vi "CHD_DRIVE_EXECUTE.vi"(6 "Pass_Through_Time":dbl=-1.0 format="%33.4f", 8 "error in (no error)":errorcluster) -> (0 "error out":errorcluster)   [LabVIEW 2019]
uses:
  <vilib>/Rock Robotics/WPI/ThirdParty/JAS_Junk/TrajLib/VI/BoolCmd_Recv_Internal.vi
  <vilib>/Rock Robotics/WPI/ThirdParty/JAS_Junk/TrajLib/VI/numCmd_Recv_Generic.vi
  <vilib>/Rock Robotics/WPI/ThirdParty/JAS_Junk/TrajLib/VI/Util_GetTime_U32.vi
  <vilib>/Rock Robotics/WPI/ThirdParty/JAS_Junk/TrajLib/MathUtil_InputModulus.vi
  <vilib>/Rock Robotics/WPI/ThirdParty/JAS_Junk/TrajLib/VI/BoolCmd_ObtainQueue.vi
  <vilib>/Rock Robotics/WPI/ThirdParty/JAS_Junk/TrajLib/VI/numCmd_ObtainQueue_Generic.vi
  CHD_DRIVE_GLOBALS.vi
  <vilib>/Rock Robotics/SystemInterfaces/Utilities/FPGA_UtilitiesRead LocalTime.vi
  <vilib>/Rock Robotics/WPI/ThirdParty/JAS_Junk/TrajLib/VI/Util_GetTime_U64.vi
  <vilib>/Rock Robotics/WPI/ThirdParty/JAS_Junk/TrajLib/Trajectory_Library.lvlib
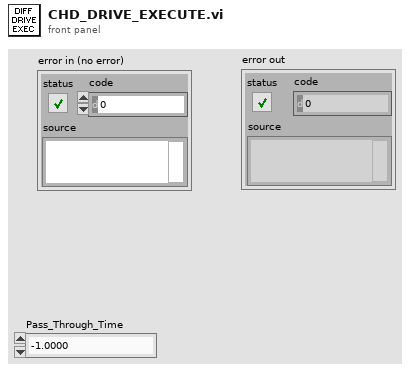
[diagram p1: front panel]
types:
  T1 = typedef "WPI_GyroDevRef.ctl" = cluster{"DevStatus":errorcluster, "Analog Channel":T2, "Gain (VoltsPerDegree/Second)":dbl, "Gyro Type":enum16{"Analog", "XRS450"}, "Handle":i32, "SPI Bus":T3, "Device Found":bool, "Sample Rate":dbl, "Calibrate On Open":bool, "Offset":dbl}
  T2 = typedef "FPGA_AIChannel.ctl" = enum8{"AI 0", "AI 1", "AI 2", "AI 3", "AI MXP 0", "AI MXP 1", "AI MXP 2", "AI MXP 3", "Invalid"}
  T3 = typedef "spi_bus.ctl" = enum16{"SPI On-Board, CS0", "SPI On-Board, CS1", "SPI On-Board, CS2", "SPI On-Board, CS3", "SPI MXP", "Invalid"}
  T4 = typedef "CHD_DRIVE_MODULE_TYPDEF.ctl" = cluster{"DiffDriveMotor":T5, "DiffDriveEnc":T10}
  T5 = typedef "WPI_MotorControlDeviceRef.ctl" = cluster{"DeviceStatus":errorcluster, "Type":T6, "PWM":cluster{"PWM Channel":T7, "DeadBand":T8}, "CAN":cluster{"Device Number":u8, "SetOutput VI Ref":variant, "GetOutput VI Ref":variant, "Enable VI Ref":variant, "Disable VI Ref":variant, "Data":variant}, "Invert":bool, "DIO PWM":cluster{"PWM \"Enable\" Channel":T7, "DIOChannel":T9, "PWM Rate":dbl}}
  T6 = typedef "WPI_MotorControlType.ctl" = enum16{"PWM", "CAN", "DIO PWM"}
  T7 = typedef "FPGA_DIOPWMChannel.ctl" = enum8{"PWM 0", "PWM 1", "PWM 2", "PWM 3", "PWM 4", "PWM 5", "PWM 6", "PWM 7", "PWM 8", "PWM 9", "PWM MXP 0", "PWM MXP 1", "PWM MXP 2", "PWM MXP 3", "PWM MXP 4", "PWM MXP 5", "PWM MXP 6", "PWM MXP 7", "PWM MXP 8", "PWM MXP 9", "Invalid"}
  T8 = typedef "WPI_PWMDeadband.ctl" = cluster{"Name":string, "maxPositivePwm":i32, "minPositivePwm":i32, "centerPwm":i32, "maxNegativePwm":i32, "minNegativePwm":i32, "angularRange":u16}
  T9 = typedef "FPGA_DIOChannel.ctl" = enum8{"DIO 0", "DIO 1", "DIO 2", "DIO 3", "DIO 4", "DIO 5", "DIO 6", "DIO 7", "DIO 8", "DIO 9", "DIO MXP 0", "DIO MXP 1", "DIO MXP 2", "DIO MXP 3", "DIO MXP 4", "DIO MXP 5", "DIO MXP 6", "DIO MXP 7", "DIO MXP 8", "DIO MXP 9", "DIO MXP 10", "DIO MXP 11", "DIO MXP 12", "DIO MXP 13", "DIO MXP 14", "DIO MXP 15", "SPI Port CS1", "SPI Port CS2", "SPI Port CS3", "SPI Port MISO", "SPI Port MOSI", "Invalid"}
  T10 = typedef "WPI_EncoderDevRef.ctl" = cluster{"DevStatus":errorcluster, "EncoderIndex":T11, "CounterIndex":T12, "DistancePerCount":dbl, "Decoding Type":T13}
  T11 = typedef "FPGA_EncoderIdx.ctl" = enum8{"Enc 0", "Enc 1", "Enc 2", "Enc 3", "Enc 4", "Enc 5", "Enc 6", "Enc 7", "Invalid"}
  T12 = typedef "FPGA_CounterCtrSystemIndex.ctl" = enum8{"Ctr 0", "Ctr 1", "Ctr 2", "Ctr 3", "Ctr 4", "Ctr 5", "Ctr 6", "Ctr 7", "Invalid"}
  T13 = typedef "WPI_EncoderType.ctl" = enum16{"1x", "2x", "4x"}
  T14 = typedef "Trajectory_Library.lvlib/DIFF_DRIVE_KINEMATICS.ctl" = cluster{"TrackWidth_Meters":dbl}
  T15 = typedef "Trajectory_Library.lvlib/CHASSIS_SPEEDS.ctl" = cluster{"vX":dbl, "vY":dbl, "vOmega":dbl}
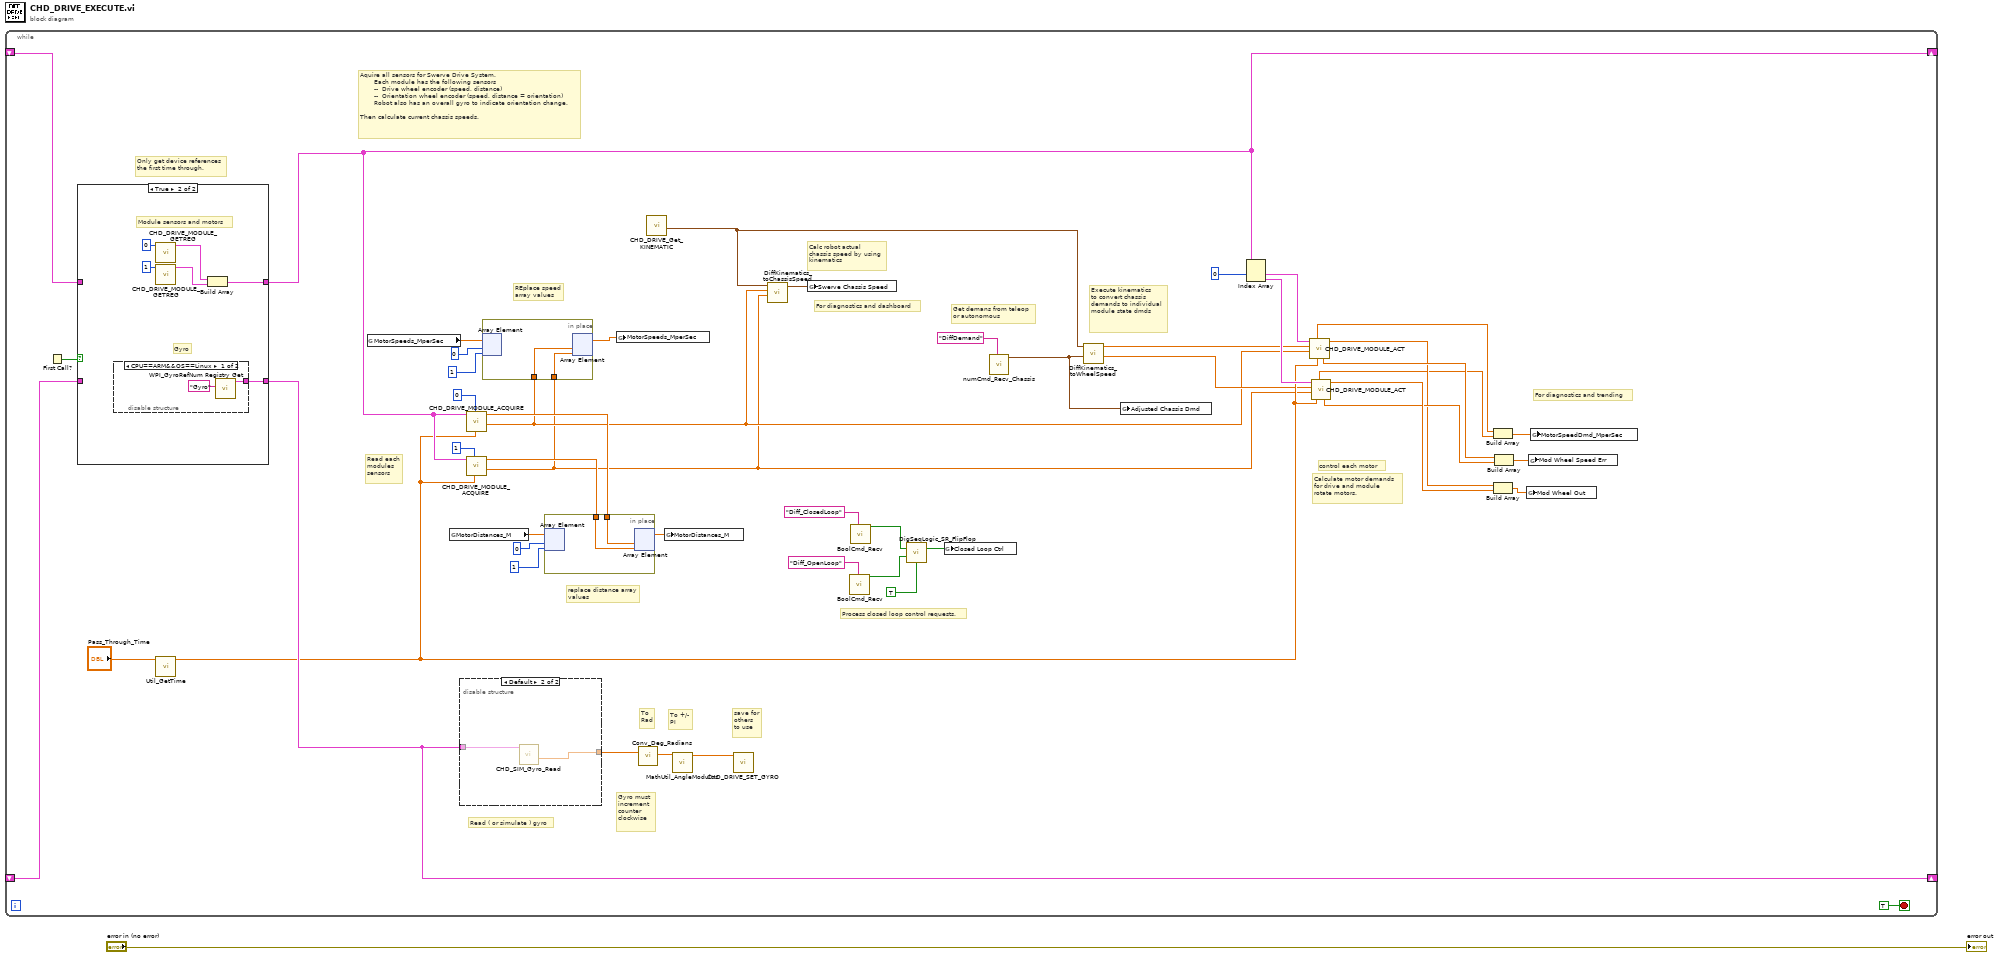
[diagram p0: block diagram]
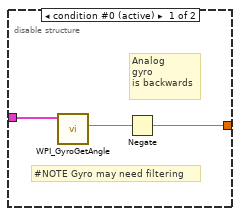
[diagram p4: hidden frame]
diagram:
  n1 = while {
    shift-right: [w29] -> _
    shift-left: _ -> [w30]
    shift-right: [w28] -> _
    shift-left: _ -> [w27]
    stop <- TRUE stop-if-true
    # "replace distance array\nvalues"
    # "REplace speed\narray values"
    # "Process closed loop control requests."
    # "Only get device references\nthe first time through."
    # "save for\nothers\nto use"
    # "For diagnostics and trending"
    # "For diagnostics and dashboard"
    # "Read each\nmodules\nsensors"
    # "Gyro must\nincrement \ncounter\nclockwise"
    # "To +/-\nPI"
    # "To\nRad"
    # "Read ( or simulate ) gyro"
    # "Aquire all sensors for Swerve Drive System.\n       Each module has the following sensors\n       --  Drive wheel encoder (speed, distance)\n       --  Orientation wheel encoder (speed, distance = orientation)\n       Robot also has an overall gyro to indicate orientation change.\n\nThen calculate current chassis speeds."
    # "Calc robot actual\nchassis speed by using\nkinematics"
    # "Calculate motor demands\nfor drive and module \nrotate motors."
    # "Execute kinematics\nto convert chassis \ndemands to individual\nmodule state dmds"
    # "Get demans from teleop\nor autonomous"
    # "control each motor"
    n2 = First Call?() -> (First Call?: T/F=w31:bool)
    n3 = case shown="True" w31 {
      tunnel: [w56 w60] -> w29
      tunnel: [w55 w59] -> w28
      tunnel: w30 -> [w56 _]
      tunnel: w27 -> [w55 _]
      frame False {
      }
      frame True {
        # "Module sensors and motors"
        # "Gyro"
        n4 = disable-structure shown="CPU==ARM&&OS==Linux" {
          disable-tunnel: [w63 _] -> w59
          frame condition #0 (active) {
            n5 = call <vilib>:"WPI_GyroRefNum Registry Get.vi"("refnum name"="Gyro") -> ("GyroDevRef"=w63:T1)  [unwired: 9 in, 1 out]
          }
          frame condition #1 {
          }
        }
        n6 = call "CHD_DRIVE_MODULE_GETREG.vi"("Suffix"=0) -> ("Diff Module TypDef"=w61:T4)  [unwired: 10 in]
        n7 = call "CHD_DRIVE_MODULE_GETREG.vi"("Suffix"=1) -> ("Diff Module TypDef"=w62:T4)  [unwired: 10 in]
        n8 = Build Array(w61, w62) -> (w60:T4[])
      }
    }
    n9 = call <vilib>:"Util_GetTime.vi"("Pass_Through_Time"="Pass_Through_Time") -> ("FPGA_Time_Seconds"=w17:dbl)  [unwired: 8 in, 2 out]
    n10 = global read "CHD_DRIVE_GLOBALS.vi" "MotorSpeeds_MperSec"() -> (w9:dbl[])
    n11 = global read "CHD_DRIVE_GLOBALS.vi" "MotorDistances_M"() -> (w6:dbl[])
    n12 = disable-structure shown="Default" {
      disable-tunnel: w28 -> [w67 w69]
      disable-tunnel: [w65 w68] -> w35
      frame condition #0 (active) {
        # "Analog\ngyro\nis backwards"
        # "#NOTE Gyro may need filtering"
        n13 = call <vilib>:"WPI_GyroGetAngle.vi"("GyroDevRef"=w67) -> ("Angle"=w66:dbl)  [unwired: 6 in, 4 out]
        n14 = Negate(x=w66) -> (-x=w65:dbl)
      }
      frame condition #1 {
        n15 = call "CHD_SIM_Gyro_Read.vi"("GyroDevRef"=w69) -> ("Gyro_Cont_Deg"=w68:dbl)  [unwired: 10 in]
      }
    }
    n16 = call "CHD_DRIVE_MODULE_ACQUIRE.vi"("Pass_Through_Time"=w17, "Swerve Module Inx"=1, "Diff Module TypDef"=w29) -> ("Speed_MPS"=w2:dbl, "Distance_M"=w11:dbl)  [unwired: 7 in]
    n17 = call "CHD_DRIVE_MODULE_ACQUIRE.vi"("Pass_Through_Time"=w17, "Swerve Module Inx"=0, "Diff Module TypDef"=w29) -> ("Speed_MPS"=w3:dbl, "Distance_M"=w12:dbl)  [unwired: 7 in]
    n18 = in-place {
      in-place-border: w3 -> [w54]
      in-place-border: w2 -> [w53]
      n19 = in-place-array #1(w9, 0, 1) -> ()  [unwired: 2 out]
      n20 = in-place-array #1(w54, w53) -> (w8:dbl[])  [unwired: 2 out]
    }
    n21 = in-place {
      in-place-border: w12 -> [w52]
      in-place-border: w11 -> [w51]
      n22 = in-place-array #2(w6, 0, 1) -> ()  [unwired: 2 out]
      n23 = in-place-array #2(w52, w51) -> (w7:dbl[])  [unwired: 2 out]
    }
    n24 = global write "CHD_DRIVE_GLOBALS.vi" "MotorSpeeds_MperSec"(w8) -> ()
    n25 = call <vilib>:"Conv_Deg_Radians.vi"("Degress"=w35) -> ("Radians"=w39:dbl)  [unwired: 10 in]
    n26 = call "CHD_DRIVE_Get_KINEMATIC.vi"() -> ("out DIFF_DRIVE_KINEMATICS"=w10:T14)  [unwired: 11 in]
    n27 = global write "CHD_DRIVE_GLOBALS.vi" "MotorDistances_M"(w7) -> ()
    n28 = call <vilib>:"MathUtil_AngleModulus.vi"("InputAngle"=w39) -> ("ModulsAngle"=w33:dbl)  [unwired: 10 in]
    n29 = call "CHD_DRIVE_SET_GYRO.vi"("Gyro Heading Radians"=w33) -> ()  [unwired: 11 in]
    n30 = call <vilib>:"DiffKinematics_toChassisSpeed.vi"("RightVelocity"=w2, "LeftVelocity"=w3, "inDIFF_DRIVE_KINEMATICS"=w10) -> ("CHASSIS Speed"=w38:T15)  [unwired: 8 in]
    n31 = global write "CHD_DRIVE_GLOBALS.vi" "Swerve Chassis Speed"(w38) -> ()
    n32 = call <vilib>:"BoolCmd_Recv.vi"("Command Name"="Diff_OpenLoop") -> ("New Request"=w20:bool)  [unwired: 9 in, 1 out]
    n33 = call <vilib>:"BoolCmd_Recv.vi"("Command Name"="Diff_ClosedLoop") -> ("New Request"=w21:bool)  [unwired: 9 in, 1 out]
    n34 = call <vilib>:"DigSeqLogic_SR_FlipFlop.vi"("Set"=w21, "Reset"=w20, "Initial Value"=TRUE) -> ("Output"=w18:bool)  [unwired: 11 in, 1 out]
    n35 = global write "CHD_DRIVE_GLOBALS.vi" "Closed Loop Ctrl"(w18) -> ()
    n36 = call <vilib>:"numCmd_Recv_Chassis.vi"("Command Name"="DiffDemand") -> ("Chassis Speeds"=w34:T15)  [unwired: 8 in, 2 out]
    n37 = call <vilib>:"DiffKinematics_toWheelSpeed.vi"("CHASSIS Speed"=w34, "DIFF_DRIVE_KINEMATICS"=w10) -> ("RightVelocity"=w4:dbl, "LeftVelocity"=w5:dbl)  [unwired: 8 in]
    n38 = global write "CHD_DRIVE_GLOBALS.vi" "Adjusted Chassis Dmd"(w34) -> ()
    n39 = Index Array(array=w29, index #1=0 ("index")) -> (element #1=w44:T4, element #2=w45:T4)  [unwired: 1 in]
    n40 = call "CHD_DRIVE_MODULE_ACT.vi"("Pass_Through_Time"=w17, "Speed Actual"=w3, "Speed Dmd"=w5, "Diff Module TypDef"=w44) -> ("Wheel Motor Dmd"=w46:dbl, "WheelSpeedErr"=w48:dbl, "Optimized Speed \nDmd M/S"=w26:dbl)  [unwired: 5 in]
    n41 = call "CHD_DRIVE_MODULE_ACT.vi"("Pass_Through_Time"=w17, "Speed Actual"=w2, "Speed Dmd"=w4, "Diff Module TypDef"=w45) -> ("Wheel Motor Dmd"=w50:dbl, "WheelSpeedErr"=w49:dbl, "Optimized Speed \nDmd M/S"=w25:dbl)  [unwired: 5 in]
    n42 = Build Array(w26, w25) -> (w24:dbl[])
    n43 = Build Array(w46, w50) -> (w43:dbl[])
    n44 = Build Array(w48, w49) -> (w42:dbl[])
    n45 = global write "CHD_DRIVE_GLOBALS.vi" "Mod Wheel Out"(w43) -> ()
    n46 = global write "CHD_DRIVE_GLOBALS.vi" "Mod Wheel Speed Err"(w42) -> ()
    n47 = global write "CHD_DRIVE_GLOBALS.vi" "MotorSpeedDmd_MperSec"(w24) -> ()
  }
  "error out" <- "error in (no error)"
